vi "Analog_multimeter.vi"() -> ()   [LabVIEW 2021]
uses:
  Controls/Enum_states.ctl
  <vilib>/Analysis/5stat.llb/RMS (DBL).vi
  Globals/CH1.vi
  Globals/CH2.vi
  Globals/CH3.vi
  Globals/CH4.vi
  Globals/CH5.vi
  <vilib>/Analysis/3filter.llb/Butterworth Filter (DBL).vi
  Globals/Global message.vi
  <vilib>/Analysis/NI_AALPro.lvlib
  <vilib>/Analysis/NI_AALBase.lvlib
panel:
  in  "Input channel":T1(ring)
  in  "Output channel":T1(ring)
  in  "Data":bool
  in  "Write":bool
  in  "Stop Button":bool
  out "Terminal GND":bool
  out "Terminal_I":bool
  out "Terminal_V":bool
  in  "Zero instrument":dbl(knob) scale=-2.0..2.0
  in  "Zero resistance":dbl(knob) scale=-1.0..1.0
  in  "Selector":i32(knob)=10 min=0 max=20 step=1 scale=0.0..20.0
  out "Main indicator":dbl(knob) max=1000.0 scale=0.0..250.0
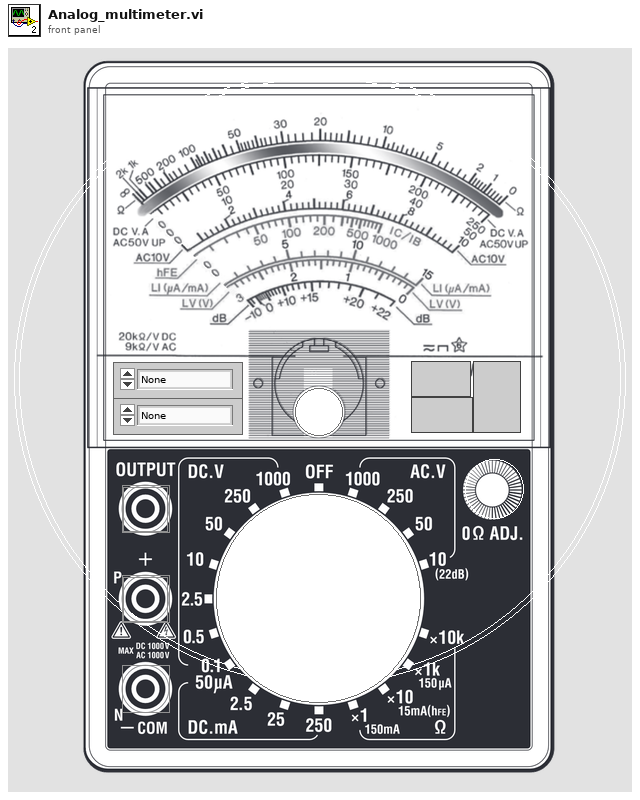
[diagram p1: front panel]
types:
  T1 = enum16{"None", "CH 1", "CH 2", "CH 3", "CH 4", "CH 5"}
  T2 = enum16{"open", "replace", "create", "open or create", "replace or create", "replace or create with confirmation"}
  T3 = typedef "Enum_states.ctl" = enum16{"Initialize", "Run", "Load", "Stop"}
  T4 = cluster{"Main indicator":dbl, "Terminal_V":bool, "Terminal_I":bool, "Terminal GND":bool, "Message":string}
  T5 = cluster{"Zero instrument":dbl, "Selector":i32, "Zero resistance":dbl}
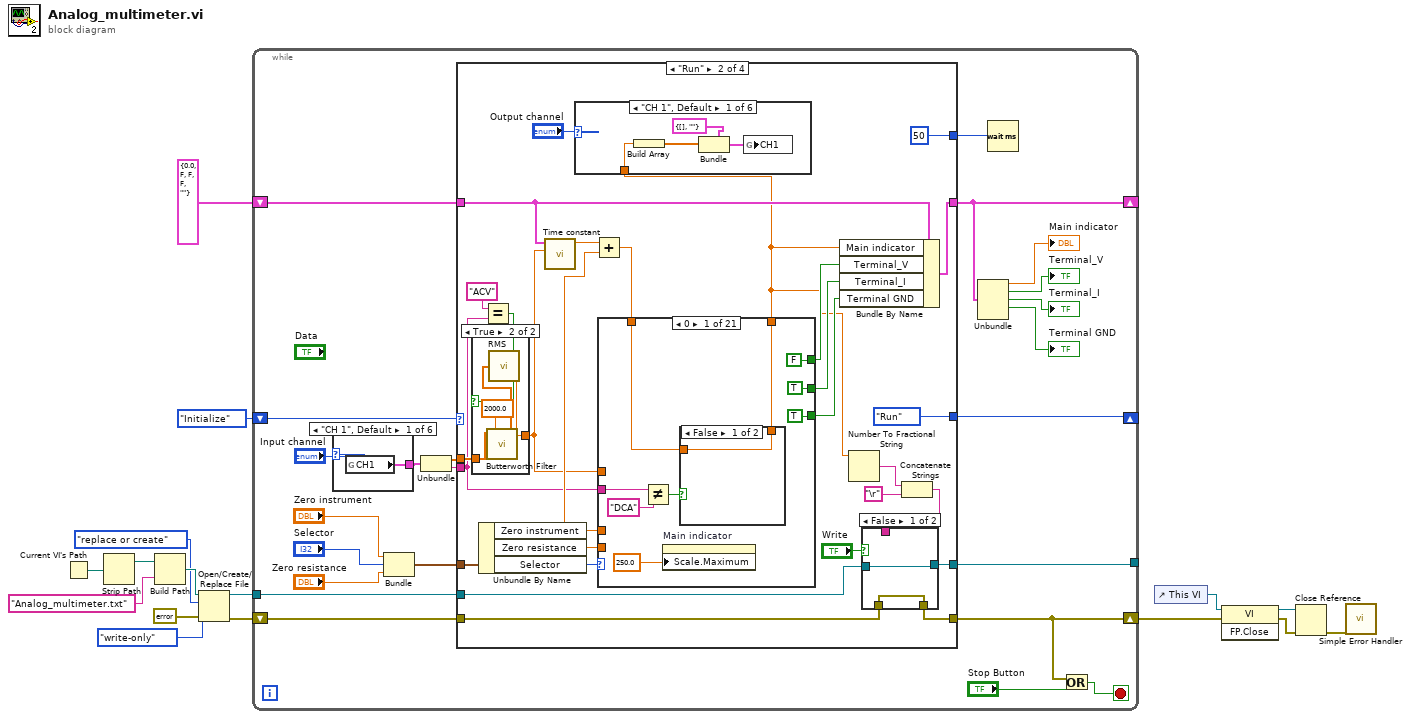
[diagram p0: block diagram]
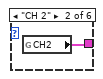
[diagram p2: hidden frame]
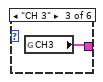
[diagram p3: hidden frame]
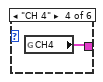
[diagram p4: hidden frame]
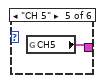
[diagram p5: hidden frame]
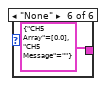
[diagram p6: hidden frame]
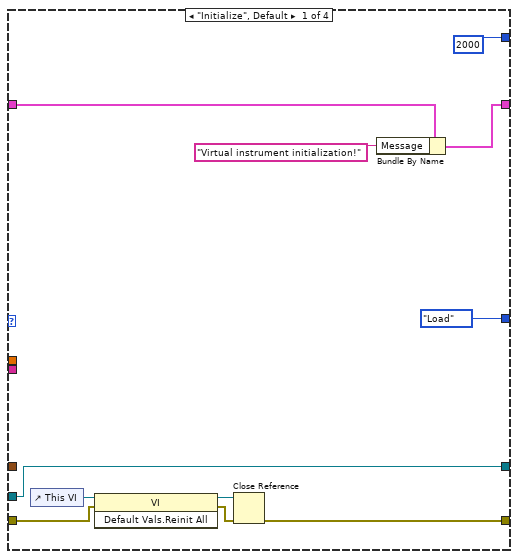
[diagram p7: hidden frame]
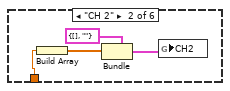
[diagram p8: hidden frame]
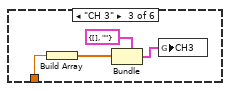
[diagram p9: hidden frame]
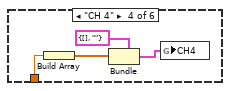
[diagram p10: hidden frame]
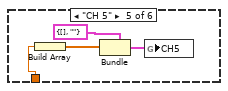
[diagram p11: hidden frame]
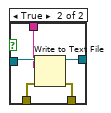
[diagram p13: hidden frame]
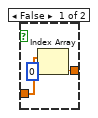
[diagram p14: hidden frame]
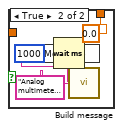
[diagram p15: hidden frame]
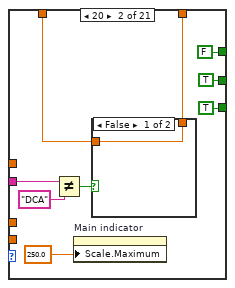
[diagram p16: hidden frame]
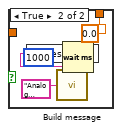
[diagram p17: hidden frame]
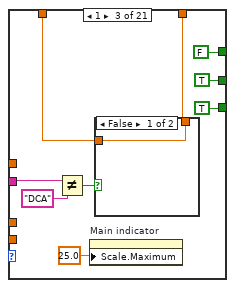
[diagram p18: hidden frame]
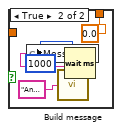
[diagram p19: hidden frame]
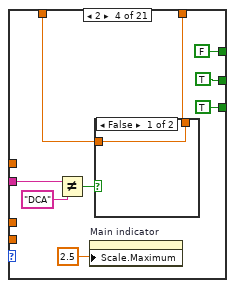
[diagram p20: hidden frame]
diagram:
  n1 = Current VI's Path() -> (path=w7:path)
  n2 = Strip Path(path=w7) -> (stripped path=w6:path)  [unwired: 1 out]
  n3 = Build Path(base path=w6, name or relative path="Analog_multimeter.txt") -> (appended path=w4:path)
  n4 = Open/Create/Replace File(file path (use dialog)=w4, error in=errorcluster {"status"=FALSE, "code"=0, "source"=""} ("error constant"), operation (0:open)=T2."replace or create", access (0:read/write)=enum16{"read/write", "read-only", "write-only"}."write-only") -> (refnum out=w1:refnum<file>, error out=w9:errorcluster)  [unwired: 2 in, 1 out]
  n5 = while {
    shift-right: [w33] -> w14
    shift-left: w9 -> [w35]
    shift-right: [w28] -> _
    shift-left: T4 {"Main indicator"=0.0, "Terminal_V"=FALSE, "Terminal_I"=FALSE, "Terminal GND"=FALSE, "Message"=""} -> [w31]
    shift-right: [w29] -> _
    shift-left: Enum_states."Initialize" ("Enum") -> [w30]
    tunnel: w1 -> [w18]
    tunnel: [w17] -> _
    stop <- w34 stop-if-true
    n6 = case shown="\"CH 1\", Default" "Input channel" {
      tunnel: [w40 w41 w42 w43 w44 cluster{"CH5 Array":dbl[], "CH5 Message":string} {"CH5 Array"=[0.0], "CH5 Message"=""} ("CH5")] -> w21
      frame "CH 1", Default {
        n7 = global read "CH1.vi" "CH1"() -> (w40:cluster{"CH1 Array":dbl[], "CH1 Message":string})
      }
      frame "CH 2" {
        n8 = global read "CH2.vi" "CH2"() -> (w41:cluster{"CH2 Array":dbl[], "CH2 Message":string})
      }
      frame "CH 3" {
        n9 = global read "CH3.vi" "CH3"() -> (w42:cluster{"CH3 Array":dbl[], "CH3 Message":string})
      }
      frame "CH 4" {
        n10 = global read "CH4.vi" "CH4"() -> (w43:cluster{"CH4 Array":dbl[], "CH4 Message":string})
      }
      frame "CH 5" {
        n11 = global read "CH5.vi" "CH5"() -> (w44:cluster{"CH5 Array":dbl[], "CH5 Message":string})
      }
      frame "None" {
      }
    }
    n12 = Bundle("Zero instrument"="Zero instrument", "Selector"="Selector", "Zero resistance"="Zero resistance") -> (w36:T5)  [unwired: 1 in]
    n13 = Unbundle(w21) -> ("CH5 Array"=w20:dbl[], "CH5 Message"=w19:string)
    n14 = case shown="\"Run\"" w30 {
      tunnel: w36 -> [_ w82 _ _]
      tunnel: w35 -> [w53 w64 w408 w410]
      tunnel: [w47 w63 w408 w410] -> w33
      tunnel: w31 -> [w49 w75 w406 _]
      tunnel: [w48 w83 w406 _] -> w28
      tunnel: [Enum_states."Load" ("Enum") Enum_states."Run" ("Enum") Enum_states."Run" ("Enum") _] -> w29
      tunnel: w20 -> [_ w71 _ _]
      tunnel: [u32 2000 ("milliseconds to wait") u32 50 ("milliseconds to wait") u32 50 ("milliseconds to wait") _] -> w23
      tunnel: w19 -> [_ w70 _ _]
      tunnel: w18 -> [w46 w65 w403 w411]
      tunnel: [w46 w59 w403 w411] -> w17
      frame "Initialize", Default {
        n15 = control-ref of="This VI"() -> (w56:refnum<vi>)
        n16 = invoke class="VI" method="Default Vals.Reinit All"(reference=w56, error in=w53) -> (reference out=w55:refnum<vi>, error out=w54:errorcluster)  [unwired: 1 in, 1 out]
        n17 = Close Reference(reference=w55, error in (no error)=w54) -> (error out=w47:errorcluster)
        n18 = Bundle By Name(cluster=w49, "Message"="Virtual instrument initialization!") -> (w48:T4)
      }
      frame "Run" {
        n19 = Unbundle By Name(w82) -> ("Zero instrument"=w73:dbl, "Zero resistance"=w77:dbl, "Selector"=w81:i32)
        n20 = Equal?(x="ACV", y=w70) -> (x = y?=w68:bool)
        n21 = case shown="True" w68 {
          tunnel: w71 -> [w113 w117]
          tunnel: [w112 w118] -> w67
          frame False {
            n22 = Index Array(array=w113, index=0) -> (element=w112:dbl)
          }
          frame True {
            n23 = call-poly <vilib>:"Butterworth Filter.vi"("high cutoff freq: fh"=2000.0, "X"=w117) -> ("Filtered X"=w116:dbl[])  [unwired: 6 in, 1 out]
            n24 = call-poly <vilib>:"RMS.vi"("X"=w116) -> ("rms value"=w118:dbl)  [unwired: 1 out]
          }
        }
        n25 = call "Time constant.vi"("Numeric in"=w67, "Cluster"=w75) -> ("Numeric out"=w74:dbl)  [unwired: 9 in]
        n26 = Add(x=w74, y=w73) -> (x+y=w72:dbl)
        n27 = case shown="0" w81 {
          tunnel: [FALSE FALSE FALSE FALSE FALSE TRUE TRUE TRUE TRUE TRUE TRUE FALSE TRUE TRUE TRUE TRUE FALSE TRUE TRUE TRUE FALSE] -> w80
          tunnel: [TRUE TRUE TRUE TRUE TRUE FALSE FALSE FALSE FALSE FALSE FALSE FALSE FALSE FALSE FALSE FALSE TRUE FALSE FALSE FALSE TRUE] -> w79
          tunnel: [TRUE TRUE TRUE TRUE TRUE TRUE TRUE TRUE TRUE TRUE TRUE FALSE TRUE TRUE TRUE TRUE TRUE TRUE TRUE TRUE TRUE] -> w78
          tunnel: w77 -> [_ _ _ _ _ _ _ _ _ _ _ _ _ _ _ _ _ _ _ _ _]
          tunnel: w73 -> [_ _ _ _ _ _ _ _ _ _ _ _ _ _ _ _ _ _ _ _ _]
          tunnel: w72 -> [w120 w134 w148 w162 w176 w190 w204 w218 w232 w246 w260 _ w278 w292 w306 w320 w334 w350 w362 w376 w390]
          tunnel: [w119 w133 w147 w161 w175 w189 w203 w217 w231 w245 w259 0.0 w277 w291 w305 w319 w333 w349 w361 w375 w389] -> w57
          tunnel: w70 -> [w123 w137 w149 w163 w177 w191 w205 w219 w233 w247 w261 _ w279 w293 w307 w321 w335 w348 w363 w377 w391]
          tunnel: w67 -> [_ _ _ _ _ _ _ _ _ _ _ _ _ _ _ _ _ _ _ _ _]
          frame 0 {
            n28 = Not Equal?(x=w123, y="DCA") -> (x != y?=w121:bool)
            n29 = property on="Main indicator" class="Knob (strict)"("Scale.Maximum"=250.0 ("Data Entry Limits:Minimum")) -> ()  [unwired: 2 in, 2 out]
            n30 = case shown="False" w121 {
              tunnel: w120 -> [w128 _]
              tunnel: [w128 0.0] -> w119
              frame False {
              }
              frame True {
                n31 = Wait (ms)(milliseconds to wait=u32 1000) -> ()  [unwired: 1 out]
                n32 = call "Build message.vi"("Input string"="Analog multimeter: wrong measurement range") -> ("Output string"=w129:string)
                n33 = global write "Global message.vi" "Message"(w129) -> ()
              }
            }
          }
          frame 20 {
            n34 = Not Equal?(x=w137, y="DCA") -> (x != y?=w135:bool)
            n35 = property on="Main indicator" class="Knob (strict)"("Scale.Maximum"=250.0 ("Data Entry Limits:Minimum")) -> ()  [unwired: 2 in, 2 out]
            n36 = case shown="False" w135 {
              tunnel: w134 -> [w142 _]
              tunnel: [w142 0.0] -> w133
              frame False {
              }
              frame True {
                n37 = call "Build message.vi"("Input string"="Analog multimeter: wrong measurement range") -> ("Output string"=w143:string)
                n38 = global write "Global message.vi" "Message"(w143) -> ()
                n39 = Wait (ms)(milliseconds to wait=u32 1000) -> ()  [unwired: 1 out]
              }
            }
          }
          frame 1 {
            n40 = Not Equal?(x=w149, y="DCA") -> (x != y?=w150:bool)
            n41 = property on="Main indicator" class="Knob (strict)"("Scale.Maximum"=25.0 ("Data Entry Limits:Minimum")) -> ()  [unwired: 2 in, 2 out]
            n42 = case shown="False" w150 {
              tunnel: w148 -> [w156 _]
              tunnel: [w156 0.0] -> w147
              frame False {
              }
              frame True {
                n43 = call "Build message.vi"("Input string"="Analog multimeter: wrong measurement range") -> ("Output string"=w157:string)
                n44 = global write "Global message.vi" "Message"(w157) -> ()
                n45 = Wait (ms)(milliseconds to wait=u32 1000) -> ()  [unwired: 1 out]
              }
            }
          }
          frame 2 {
            n46 = Not Equal?(x=w163, y="DCA") -> (x != y?=w164:bool)
            n47 = property on="Main indicator" class="Knob (strict)"("Scale.Maximum"=2.5 ("Data Entry Limits:Minimum")) -> ()  [unwired: 2 in, 2 out]
            n48 = case shown="False" w164 {
              tunnel: w162 -> [w170 _]
              tunnel: [w170 0.0] -> w161
              frame False {
              }
              frame True {
                n49 = call "Build message.vi"("Input string"="Analog multimeter: wrong measurement range") -> ("Output string"=w171:string)
                n50 = global write "Global message.vi" "Message"(w171) -> ()
                n51 = Wait (ms)(milliseconds to wait=u32 1000) -> ()  [unwired: 1 out]
              }
            }
          }
          frame 3 {
            n52 = Not Equal?(x=w177, y="DCA") -> (x != y?=w178:bool)
            n53 = property on="Main indicator" class="Knob (strict)"("Scale.Maximum"=0.1 ("Data Entry Limits:Minimum")) -> ()  [unwired: 2 in, 2 out]
            n54 = case shown="False" w178 {
              tunnel: w176 -> [w184 _]
              tunnel: [w184 0.0] -> w175
              frame False {
              }
              frame True {
                n55 = call "Build message.vi"("Input string"="Analog multimeter: wrong measurement range") -> ("Output string"=w185:string)
                n56 = global write "Global message.vi" "Message"(w185) -> ()
                n57 = Wait (ms)(milliseconds to wait=u32 1000) -> ()  [unwired: 1 out]
              }
            }
          }
          frame 4 {
            n58 = Not Equal?(x=w191, y="DCV") -> (x != y?=w192:bool)
            n59 = property on="Main indicator" class="Knob (strict)"("Scale.Maximum"=0.5 ("Data Entry Limits:Minimum")) -> ()  [unwired: 2 in, 2 out]
            n60 = case shown="False" w192 {
              tunnel: w190 -> [w198 _]
              tunnel: [w198 0.0] -> w189
              frame False {
              }
              frame True {
                n61 = call "Build message.vi"("Input string"="Analog multimeter: wrong measurement range") -> ("Output string"=w199:string)
                n62 = global write "Global message.vi" "Message"(w199) -> ()
                n63 = Wait (ms)(milliseconds to wait=u32 1000) -> ()  [unwired: 1 out]
              }
            }
          }
          frame 5 {
            n64 = Not Equal?(x=w205, y="DCV") -> (x != y?=w206:bool)
            n65 = property on="Main indicator" class="Knob (strict)"("Scale.Maximum"=2.5 ("Data Entry Limits:Minimum")) -> ()  [unwired: 2 in, 2 out]
            n66 = case shown="False" w206 {
              tunnel: w204 -> [w212 _]
              tunnel: [w212 0.0] -> w203
              frame False {
              }
              frame True {
                n67 = call "Build message.vi"("Input string"="Analog multimeter: wrong measurement range") -> ("Output string"=w213:string)
                n68 = global write "Global message.vi" "Message"(w213) -> ()
                n69 = Wait (ms)(milliseconds to wait=u32 1000) -> ()  [unwired: 1 out]
              }
            }
          }
          frame 6 {
            n70 = Not Equal?(x=w219, y="DCV") -> (x != y?=w220:bool)
            n71 = property on="Main indicator" class="Knob (strict)"("Scale.Maximum"=10.0 ("Data Entry Limits:Minimum")) -> ()  [unwired: 2 in, 2 out]
            n72 = case shown="False" w220 {
              tunnel: w218 -> [w226 _]
              tunnel: [w226 0.0] -> w217
              frame False {
              }
              frame True {
                n73 = call "Build message.vi"("Input string"="Analog multimeter: wrong measurement range") -> ("Output string"=w227:string)
                n74 = global write "Global message.vi" "Message"(w227) -> ()
                n75 = Wait (ms)(milliseconds to wait=u32 1000) -> ()  [unwired: 1 out]
              }
            }
          }
          frame 7 {
            n76 = Not Equal?(x=w233, y="DCV") -> (x != y?=w234:bool)
            n77 = property on="Main indicator" class="Knob (strict)"("Scale.Maximum"=50.0 ("Data Entry Limits:Minimum")) -> ()  [unwired: 2 in, 2 out]
            n78 = case shown="False" w234 {
              tunnel: w232 -> [w240 _]
              tunnel: [w240 0.0] -> w231
              frame False {
              }
              frame True {
                n79 = call "Build message.vi"("Input string"="Analog multimeter: wrong measurement range") -> ("Output string"=w241:string)
                n80 = global write "Global message.vi" "Message"(w241) -> ()
                n81 = Wait (ms)(milliseconds to wait=u32 1000) -> ()  [unwired: 1 out]
              }
            }
          }
          frame 8 {
            n82 = Not Equal?(x=w247, y="DCV") -> (x != y?=w248:bool)
            n83 = property on="Main indicator" class="Knob (strict)"("Scale.Maximum"=250.0 ("Data Entry Limits:Minimum")) -> ()  [unwired: 2 in, 2 out]
            n84 = case shown="False" w248 {
              tunnel: w246 -> [w254 _]
              tunnel: [w254 0.0] -> w245
              frame False {
              }
              frame True {
                n85 = call "Build message.vi"("Input string"="Analog multimeter: wrong measurement range") -> ("Output string"=w255:string)
                n86 = global write "Global message.vi" "Message"(w255) -> ()
                n87 = Wait (ms)(milliseconds to wait=u32 1000) -> ()  [unwired: 1 out]
              }
            }
          }
          frame 9 {
            n88 = Not Equal?(x=w261, y="DCV") -> (x != y?=w262:bool)
            n89 = property on="Main indicator" class="Knob (strict)"("Scale.Maximum"=1000.0 ("Data Entry Limits:Minimum")) -> ()  [unwired: 2 in, 2 out]
            n90 = case shown="False" w262 {
              tunnel: w260 -> [w268 _]
              tunnel: [w268 0.0] -> w259
              frame False {
              }
              frame True {
                n91 = call "Build message.vi"("Input string"="Analog multimeter: wrong measurement range") -> ("Output string"=w269:string)
                n92 = global write "Global message.vi" "Message"(w269) -> ()
                n93 = Wait (ms)(milliseconds to wait=u32 1000) -> ()  [unwired: 1 out]
              }
            }
          }
          frame 10, Default {
          }
          frame 11 {
            n94 = Not Equal?(x=w279, y="ACV") -> (x != y?=w280:bool)
            n95 = property on="Main indicator" class="Knob (strict)"("Scale.Maximum"=1000.0 ("Data Entry Limits:Minimum")) -> ()  [unwired: 2 in, 2 out]
            n96 = case shown="False" w280 {
              tunnel: w278 -> [w286 _]
              tunnel: [w286 0.0] -> w277
              frame False {
              }
              frame True {
                n97 = call "Build message.vi"("Input string"="Analog multimeter: wrong measurement range") -> ("Output string"=w287:string)
                n98 = global write "Global message.vi" "Message"(w287) -> ()
                n99 = Wait (ms)(milliseconds to wait=u32 1000) -> ()  [unwired: 1 out]
              }
            }
          }
          frame 12 {
            n100 = Not Equal?(x=w293, y="ACV") -> (x != y?=w294:bool)
            n101 = case shown="False" w294 {
              tunnel: w292 -> [w300 _]
              tunnel: [w300 0.0] -> w291
              frame False {
              }
              frame True {
                n102 = call "Build message.vi"("Input string"="Analog multimeter: wrong measurement range") -> ("Output string"=w301:string)
                n103 = global write "Global message.vi" "Message"(w301) -> ()
                n104 = Wait (ms)(milliseconds to wait=u32 1000) -> ()  [unwired: 1 out]
              }
            }
            n105 = property on="Main indicator" class="Knob (strict)"("Scale.Maximum"=250.0 ("Data Entry Limits:Minimum")) -> ()  [unwired: 2 in, 2 out]
          }
          frame 13 {
            n106 = Not Equal?(x=w307, y="ACV") -> (x != y?=w308:bool)
            n107 = property on="Main indicator" class="Knob (strict)"("Scale.Maximum"=50.0 ("Data Entry Limits:Minimum")) -> ()  [unwired: 2 in, 2 out]
            n108 = case shown="False" w308 {
              tunnel: w306 -> [w314 _]
              tunnel: [w314 0.0] -> w305
              frame False {
              }
              frame True {
                n109 = call "Build message.vi"("Input string"="Analog multimeter: wrong measurement range") -> ("Output string"=w315:string)
                n110 = global write "Global message.vi" "Message"(w315) -> ()
                n111 = Wait (ms)(milliseconds to wait=u32 1000) -> ()  [unwired: 1 out]
              }
            }
          }
          frame 14 {
            n112 = Not Equal?(x=w321, y="ACV") -> (x != y?=w322:bool)
            n113 = case shown="False" w322 {
              tunnel: w320 -> [w328 _]
              tunnel: [w328 0.0] -> w319
              frame False {
              }
              frame True {
                n114 = call "Build message.vi"("Input string"="Analog multimeter: wrong measurement range") -> ("Output string"=w329:string)
                n115 = global write "Global message.vi" "Message"(w329) -> ()
                n116 = Wait (ms)(milliseconds to wait=u32 1000) -> ()  [unwired: 1 out]
              }
            }
            n117 = property on="Main indicator" class="Knob (strict)"("Scale.Maximum"=10.0 ("Data Entry Limits:Minimum")) -> ()  [unwired: 2 in, 2 out]
          }
          frame 15 {
            n118 = Not Equal?(x=w335, y="DCA") -> (x != y?=w336:bool)
            n119 = case shown="False" w336 {
              tunnel: w334 -> [w342 _]
              tunnel: [w342 0.0] -> w333
              frame False {
              }
              frame True {
                n120 = call "Build message.vi"("Input string"="Analog multimeter: wrong measurement range") -> ("Output string"=w343:string)
                n121 = global write "Global message.vi" "Message"(w343) -> ()
                n122 = Wait (ms)(milliseconds to wait=u32 1000) -> ()  [unwired: 1 out]
              }
            }
            n123 = property on="Main indicator" class="Knob (strict)"("Scale.Maximum"=10.0 ("Data Entry Limits:Minimum")) -> ()  [unwired: 2 in, 2 out]
          }
          frame 16 {
            n124 = Not Equal?(x=w348, y="R") -> (x != y?=w351:bool)
            n125 = property on="Main indicator" class="Knob (strict)"("Scale.Maximum"=20000000.0 ("Data Entry Limits:Minimum")) -> ()  [unwired: 2 in, 2 out]
            n126 = case shown="False" w351 {
              tunnel: w350 -> [w356 _]
              tunnel: [w356 0.0] -> w349
              frame False {
              }
              frame True {
                n127 = call "Build message.vi"("Input string"="Analog multimeter: wrong measurement range") -> ("Output string"=w357:string)
                n128 = global write "Global message.vi" "Message"(w357) -> ()
                n129 = Wait (ms)(milliseconds to wait=u32 1000) -> ()  [unwired: 1 out]
              }
            }
          }
          frame 17 {
            n130 = Not Equal?(x=w363, y="R") -> (x != y?=w365:bool)
            n131 = case shown="False" w365 {
              tunnel: w362 -> [w370 _]
              tunnel: [w370 0.0] -> w361
              frame False {
              }
              frame True {
                n132 = call "Build message.vi"("Input string"="Analog multimeter: wrong measurement range") -> ("Output string"=w371:string)
                n133 = global write "Global message.vi" "Message"(w371) -> ()
                n134 = Wait (ms)(milliseconds to wait=u32 1000) -> ()  [unwired: 1 out]
              }
            }
            n135 = property on="Main indicator" class="Knob (strict)"("Scale.Maximum"=2000000.0 ("Data Entry Limits:Minimum")) -> ()  [unwired: 2 in, 2 out]
          }
          frame 18 {
            n136 = Not Equal?(x=w377, y="R") -> (x != y?=w379:bool)
            n137 = case shown="False" w379 {
              tunnel: w376 -> [w384 _]
              tunnel: [w384 0.0] -> w375
              frame False {
              }
              frame True {
                n138 = call "Build message.vi"("Input string"="Analog multimeter: wrong measurement range") -> ("Output string"=w385:string)
                n139 = global write "Global message.vi" "Message"(w385) -> ()
                n140 = Wait (ms)(milliseconds to wait=u32 1000) -> ()  [unwired: 1 out]
              }
            }
            n141 = property on="Main indicator" class="Knob (strict)"("Scale.Maximum"=20000.0 ("Data Entry Limits:Minimum")) -> ()  [unwired: 2 in, 2 out]
          }
          frame 19 {
            n142 = Not Equal?(x=w391, y="R") -> (x != y?=w393:bool)
            n143 = case shown="False" w393 {
              tunnel: w390 -> [w398 _]
              tunnel: [w398 0.0] -> w389
              frame False {
              }
              frame True {
                n144 = call "Build message.vi"("Input string"="Analog multimeter: wrong measurement range") -> ("Output string"=w399:string)
                n145 = global write "Global message.vi" "Message"(w399) -> ()
                n146 = Wait (ms)(milliseconds to wait=u32 1000) -> ()  [unwired: 1 out]
              }
            }
            n147 = property on="Main indicator" class="Knob (strict)"("Scale.Maximum"=2000.0 ("Data Entry Limits:Minimum")) -> ()  [unwired: 2 in, 2 out]
          }
        }
        n148 = case shown="\"CH 1\", Default" "Output channel" {
          tunnel: w57 -> [w85 w89 w93 w97 w101 _]
          frame "CH 1", Default {
            n149 = Build Array(w85) -> (w88:dbl[])
            n150 = Bundle(cluster=cluster{"CH1 Array":dbl[], "CH1 Message":string} {"CH1 Array"=[], "CH1 Message"=""} ("CH1"), "CH1 Array"=w88) -> (w86:cluster{"CH1 Array":dbl[], "CH1 Message":string})  [unwired: 1 in]
            n151 = global write "CH1.vi" "CH1"(w86) -> ()
          }
          frame "CH 2" {
            n152 = Build Array(w89) -> (w92:dbl[])
            n153 = Bundle(cluster=cluster{"CH2 Array":dbl[], "CH2 Message":string} {"CH2 Array"=[], "CH2 Message"=""} ("CH2"), "CH2 Array"=w92) -> (w90:cluster{"CH2 Array":dbl[], "CH2 Message":string})  [unwired: 1 in]
            n154 = global write "CH2.vi" "CH2"(w90) -> ()
          }
          frame "CH 3" {
            n155 = Build Array(w93) -> (w96:dbl[])
            n156 = Bundle(cluster=cluster{"CH3 Array":dbl[], "CH3 Message":string} {"CH3 Array"=[], "CH3 Message"=""} ("CH3"), "CH3 Array"=w96) -> (w94:cluster{"CH3 Array":dbl[], "CH3 Message":string})  [unwired: 1 in]
            n157 = global write "CH3.vi" "CH3"(w94) -> ()
          }
          frame "CH 4" {
            n158 = Build Array(w97) -> (w100:dbl[])
            n159 = Bundle(cluster=cluster{"CH4 Array":dbl[], "CH4 Message":string} {"CH4 Array"=[], "CH4 Message"=""} ("CH4"), "CH4 Array"=w100) -> (w98:cluster{"CH4 Array":dbl[], "CH4 Message":string})  [unwired: 1 in]
            n160 = global write "CH4.vi" "CH4"(w98) -> ()
          }
          frame "CH 5" {
            n161 = Build Array(w101) -> (w102:dbl[])
            n162 = Bundle(cluster=cluster{"CH5 Array":dbl[], "CH5 Message":string} {"CH5 Array"=[], "CH5 Message"=""} ("CH5"), "CH5 Array"=w102) -> (w104:cluster{"CH5 Array":dbl[], "CH5 Message":string})  [unwired: 1 in]
            n163 = global write "CH5.vi" "CH5"(w104) -> ()
          }
          frame "None" {
          }
        }
        n164 = Bundle By Name(cluster=w75, "Main indicator"=w57, "Terminal_V"=w80, "Terminal_I"=w79, "Terminal GND"=w78) -> (w83:T4)
        n165 = Number To Fractional String(number=w57) -> (F-format string=w62:string)  [unwired: 3 in]
        n166 = Concatenate Strings(w62, "\r") -> (w60:string)
        n167 = case shown="False" "Write" {
          tunnel: w65 -> [w105 w111]
          tunnel: w64 -> [w106 w110]
          tunnel: [w106 w109] -> w63
          tunnel: w60 -> [_ w108]
          tunnel: [w105 w107] -> w59
          frame False {
          }
          frame True {
            n168 = Write to Text File(file (use dialog)=w111, text=w108, error in=w110) -> (refnum out=w107:refnum<file>, error out=w109:errorcluster)  [unwired: 1 in, 1 out]
          }
        }
      }
      frame "Load" {
        n169 = call "Build message.vi"("Input string"="Analog multimeter: Instrument turned OFF.\nSelect a measurement range!") -> ("Output string"=w405:string)
        n170 = global write "Global message.vi" "Message"(w405) -> ()
      }
      frame "Stop" {
      }
    }
    n171 = Unbundle(w28) -> ("Main indicator"=→"Main indicator":dbl, "Terminal_V"=→"Terminal_V":bool, "Terminal_I"=→"Terminal_I":bool, "Terminal GND"=→"Terminal GND":bool)  [unwired: 1 out]
    n172 = Wait (ms)(milliseconds to wait=w23) -> ()  [unwired: 1 out]
    n173 = Or(x=w33, y="Stop Button") -> (x .or. y?=w34:bool)
  }
  n174 = control-ref of="This VI"() -> (w12:refnum<vi>)
  n175 = invoke class="VI" method="FP.Close"(reference=w12, error in=w14) -> (reference out=w10:refnum<vi>, error out=w11:errorcluster)  [unwired: 1 in, 1 out]
  n176 = Close Reference(reference=w10, error in (no error)=w11) -> (error out=w13:errorcluster)
  n177 = call <vilib>:"Simple Error Handler.vi"("error in (no error)"=w13) -> ()  [unwired: 4 in, 5 out]
